vi "atcs_monitorCommand_Target.vi"(8 "error in (no error)":errorcluster, 11 "command_Target_Ctl":T1) -> (0 "error out":errorcluster, 2 "function return":i32, 3 "command_Target_Ctl out":T1)   [LabVIEW 2016, in "SALLV_atcs.lvlib"]
doc: "int atcs_shm_monitorCommand_TargetLV(atcs_command_TargetLV *command_Target_Ctl );"
uses:
  SALLV_atcs.lvlib
  DataTypes/command_Target.ctl
  SALLV_atcs.so
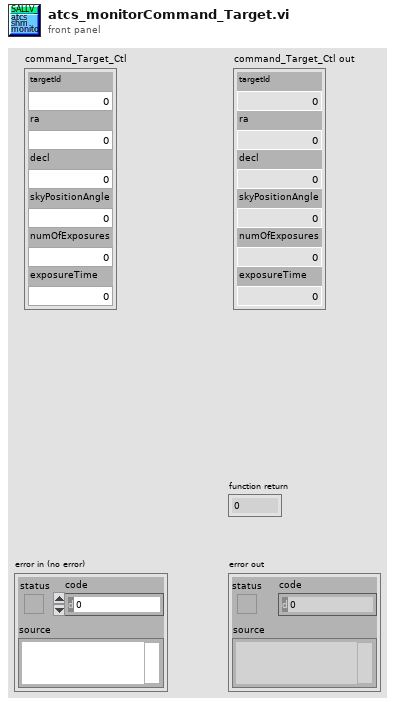
[diagram p1: front panel]
types:
  T1 = typedef "SALLV_atcs.lvlib/command_Target.ctl" = cluster{"targetId":i32, "ra":dbl, "decl":dbl, "skyPositionAngle":dbl, "numOfExposures":i32, "exposureTime":dbl}
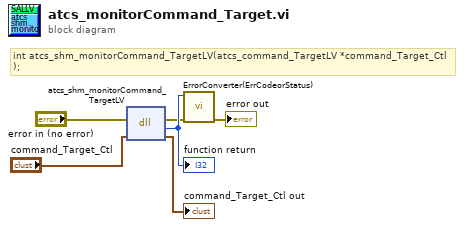
[diagram p0: block diagram]
diagram:
  # "int atcs_shm_monitorCommand_TargetLV(atcs_command_TargetLV *command_Target_Ctl );"
  n1 = dll-call lib="home/andres/Desktop/SALLV_atcs/SALLV_atcs.*" fn="atcs_shm_monitorCommand_TargetLV"(error in="error in (no error)", "command_Target_Ctl"="command_Target_Ctl") -> (error out=w2:errorcluster, w6:i32, "command_Target_Ctl"=→"command_Target_Ctl out":T1)  [unwired: 2 in, 1 out]
  "function return" <- w6
  n2 = call "ErrorConverter(ErrCodeorStatus).vi"("error in (no error)"=w2, "error code"=w6) -> ("error out"=→"error out":errorcluster)  [unwired: 9 in]
